vi "Set_PS1_Volts.vi"(6 "Current Limit (0)":dbl=0.75 min=0.0 max=6.0 format="%#.2g", 7 "Maximum Output Voltage (31)":dbl=31.0 min=0.0 max=31.0 format="%#.2f", 8 "error in":errorcluster, 9 "Output on/off":bool=TRUE, 10 "delay (secs)":dbl=0.5 format="%#_13g", 11 "Output Voltage":dbl format="%#_13g") -> (0 "error out":errorcluster, 2 "COM Port":string, 3 "Application Dir":path)   [LabVIEW 2015]
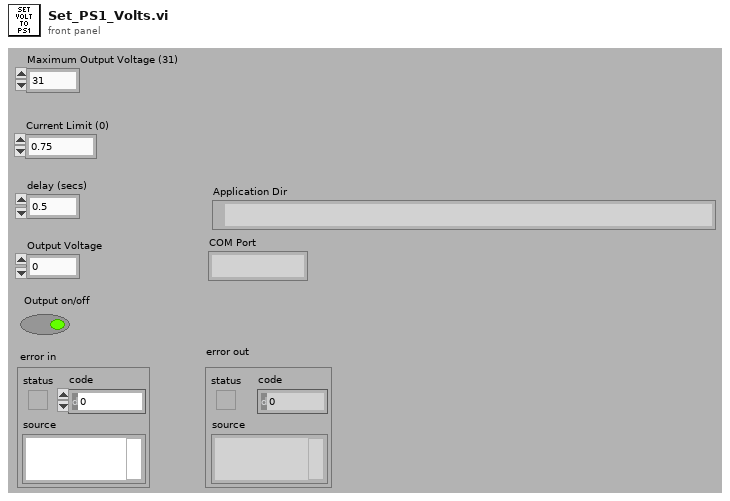
[diagram p1: front panel]
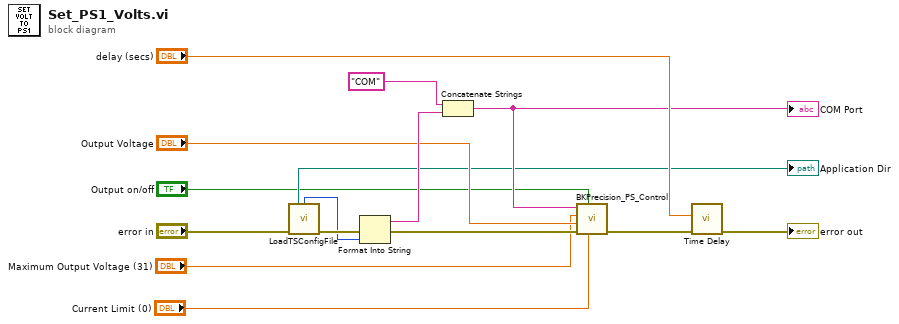
[diagram p0: block diagram]
diagram:
  n1 = call "LoadTSConfigFile.vi"("error in (no error)"="error in") -> ("appended path"=→"Application Dir":path, "PS1_COMPort"=w5:i32, "error out"=w15:errorcluster)  [unwired: 4 in, 8 out]
  n2 = Format Into String(error in=w15, w5) -> (resulting string=w13:string, error out=w7:errorcluster)  [unwired: 2 in]
  n3 = Concatenate Strings("COM" ("string"), w13) -> (w9:string)
  "COM Port" <- w9
  n4 = call "BKPrecision_PS_Control.vi"("Current Limit (0)"="Current Limit (0)", "Output on/off"="Output on/off", "error in (no error)"=w7, "Output Voltage (0)"="Output Voltage", "Maximum Output Voltage (31)"="Maximum Output Voltage (31)", "VISA resource name"=w9) -> ("error out"=w6:errorcluster)  [unwired: 4 in, 1 out]
  n5 = call "Time Delay"("error in (no error)"=w6, "Delay Time (s)"="delay (secs)") -> ("error out"=→"error out":errorcluster)  [unwired: 9 in]
